vi "Get Temperature Offset.vi"(8 "error in (no error)":errorcluster, 11 "VISA resource name":refnum<visa-resource-name>) -> (0 "error out":errorcluster, 1 "Temperature Units":i32, 2 "Temperature Offset":dbl format="%.4f", 3 "VISA resource name out":refnum<visa-resource-name>)   [LabVIEW 2014, in "Fluke 5XXX Series Multicalibrators.lvlib"]
doc: "This VI returns the temperature offset used for thermocouple measurements (±500 °C).\n\nNote:\n\nThis VI is available only for instrument models 5500A and 5520A."
uses:
  Fluke 5XXX Series Multicalibrators.lvlib
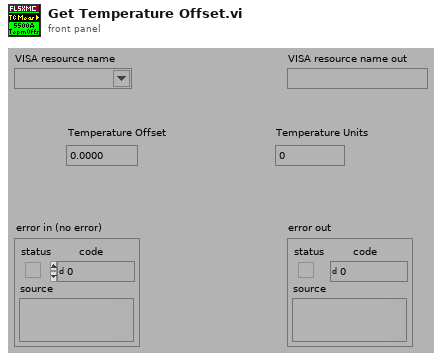
[diagram p1: front panel]
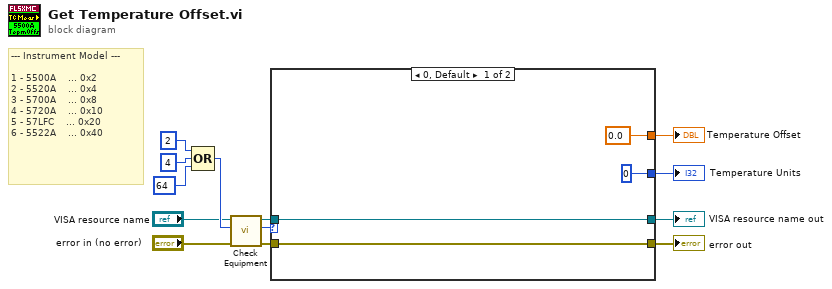
[diagram p0: block diagram]
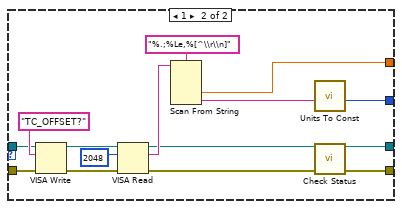
[diagram p2: hidden frame]
diagram:
  # "--- Instrument Model ---\n\n1 - 5500A    ... 0x2\n2 - 5520A    ... 0x4\n3 - 5700A    ... 0x8\n4 - 5720A    ... 0x10\n5 - 57LFC    ... 0x20\n6 - 5522A    ... 0x40"
  n1 = Compound Arithmetic op=OR(2 ("Numeric"), 4 ("Numeric"), 64 ("Numeric")) -> (w9:i32)
  n2 = call "Check Equipment.vi"("error in (no error)"="error in (no error)", "Bit Mask"=w9, "VISA resource name"="VISA resource name") -> ("error out"=w13:errorcluster, "Present?"=w12:u32, "VISA resource name out"=w11:refnum<visa-resource-name>)  [unwired: 6 in]
  n3 = case shown="0, Default" w12 {
    tunnel: [w17 w26] -> w6
    tunnel: [w16 w25] -> w5
    tunnel: w13 -> [w17 w28]
    tunnel: w11 -> [w16 w27]
    tunnel: [0 ("Index") w22] -> w4
    tunnel: [0.0 w18] -> w2
    frame 0, Default {
    }
    frame 1 {
      n4 = VISA Write(VISA resource name=w27, write buffer="TC_OFFSET?", error in (no error)=w28) -> (VISA resource name out=w31:refnum<visa-resource-name>, error out=w30:errorcluster)  [unwired: 1 out]
      n5 = VISA Read(VISA resource name=w31, byte count=u32 2048 ("byte count (0)"), error in (no error)=w30) -> (VISA resource name out=w19:refnum<visa-resource-name>, read buffer=w23:string, error out=w20:errorcluster)  [unwired: 1 out]
      n6 = Scan From String(format string="%.;%Le,%[^\\r\\n]", input string=w23) -> (output 1=w18:dbl, output 2=w21:string)  [unwired: 4 in, 3 out]
      n7 = call "Units To Const.vi"("Units"=w21) -> ("Const"=w22:i32)  [unwired: 10 in]
      n8 = call "Check Status.vi"("VISA resource name"=w19, "error in (no error)"=w20) -> ("VISA resource name out"=w25:refnum<visa-resource-name>, "error out"=w26:errorcluster)  [unwired: 12 in]
    }
  }
  "Temperature Offset" <- w2
  "Temperature Units" <- w4
  "VISA resource name out" <- w5
  "error out" <- w6
